vi "Save or Recall Instrument Setup.vi"(8 "error in (no error)":errorcluster, 9 "Memory Location (1)":u32=1, 10 "Memory Operation (0: Save)":u16(ring) items=["Save", "Recall"], 11 "VISA resource name":refnum<visa-resource-name>) -> (0 "error out":errorcluster, 3 "VISA resource name out":refnum<visa-resource-name>)   [LabVIEW 2018, in "Keithley 24XX.lvlib"]
doc: "Load a setup from or save a setup to one of the instrument's 100 slots in memory. These setups can be used for memory sweeps as well as merely storing setups for future use."
uses:
  Keithley 24XX.lvlib
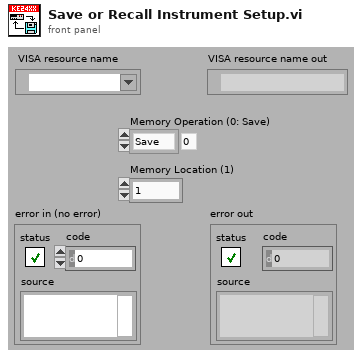
[diagram p1: front panel]
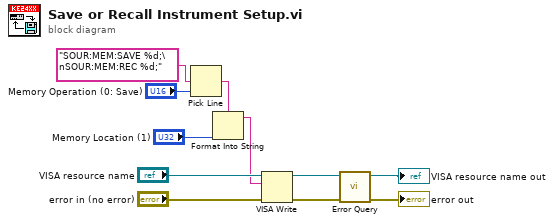
[diagram p0: block diagram]
diagram:
  n1 = Pick Line(multi-line string="SOUR:MEM:SAVE %d;\nSOUR:MEM:REC %d;" ("format string"), line index="Memory Operation (0: Save)") -> (output string=w3:string)  [unwired: 1 in]
  n2 = Format Into String(format string=w3, "Memory Location (1)") -> (resulting string=w4:string)  [unwired: 2 in, 1 out]
  n3 = VISA Write(VISA resource name="VISA resource name", write buffer=w4, error in (no error)="error in (no error)") -> (VISA resource name out=w9:refnum<visa-resource-name>, error out=w6:errorcluster)  [unwired: 1 out]
  n4 = call "Error Query.vi"("error in (no error)"=w6, "VISA resource name"=w9) -> ("error out"=→"error out":errorcluster, "VISA resource name out"=→"VISA resource name out":refnum<visa-resource-name>)  [unwired: 6 in, 2 out]
